vi "Append FFT block.vi"(8 "error in (no error)":errorcluster, 10 "new data":dbl[][](array[numeric]), 11 "ScopeBase in":refnum<class "ScopeBase.lvclass">) -> (0 "error out":errorcluster, 2 "FFT buffer":dbl[][](array[numeric]), 3 "ScopeBase out":refnum<class "ScopeBase.lvclass">)   [LabVIEW 2018, in "ScopeBase.lvclass"]
uses:
  ScopeBase.lvclass
  ScopeBase.lvclass/ScopeBase.ctl
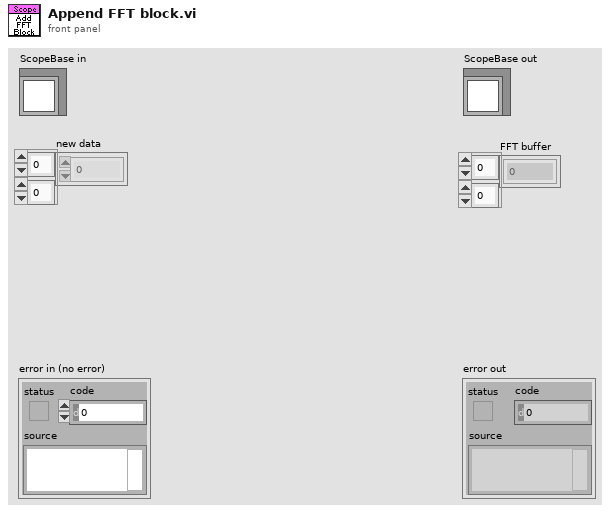
[diagram p1: front panel]
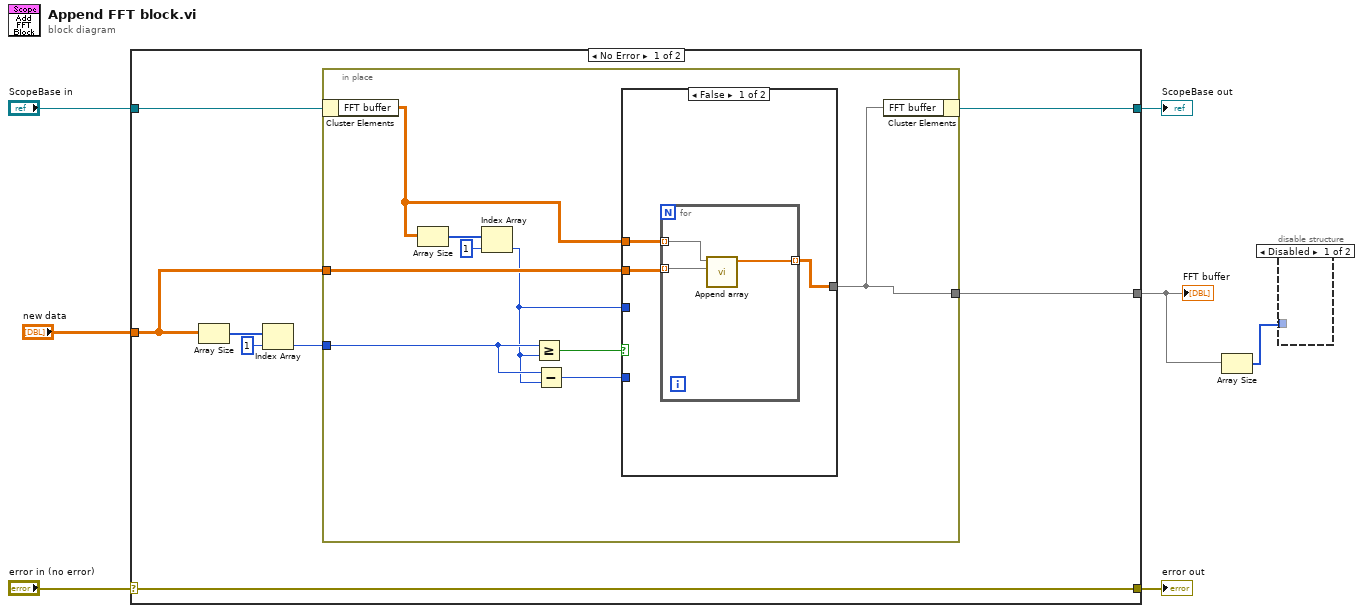
[diagram p0: block diagram]
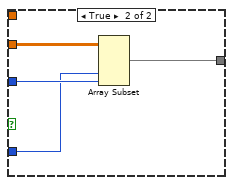
[diagram p3: hidden frame]
diagram:
  n1 = case shown="No Error" "error in (no error)" {
    selector: "error in (no error)" -> [w15 w36]
    tunnel: [w15 w36] -> w6
    tunnel: [w10 w35] -> w4
    tunnel: "ScopeBase in" -> [w13 w35]
    tunnel: "new data" -> [w9 _]
    tunnel: [w8 _] -> w2
    frame No Error {
      n2 = Array Size(array=w9) -> (size(s)=w14:i32[])
      n3 = Index Array(array=w14, index=1) -> (element=w11:i32)
      n4 = in-place {
        in-place-border: w11 -> [w20]
        in-place-border: w9 -> [w21]
        in-place-border: [w16] -> w8
        n5 = in-place-cluster #1(w13) -> ("FFT buffer"=w17:dbl[][])
        n6 = Array Size(array=w17) -> (size(s)=w24:i32[])
        n7 = Index Array(array=w24, index=1) -> (element=w19:i32)
        n8 = Greater Or Equal?(x=w20, y=w19) -> (x >= y?=w22:bool)
        n9 = Subtract(x=w20, y=w19) -> (x-y=w18:i32)
        n10 = case shown="False" w22 {
          tunnel: w21 -> [w27 w34]
          tunnel: w19 -> [_ w33]
          tunnel: w18 -> [_ w32]
          tunnel: [w25 w31] -> w16
          tunnel: w17 -> [w26 _]
          frame False {
            n11 = for {
              tunnel: w27 -> [w30] mode=indexing
              tunnel: w26 -> [w29] mode=indexing
              tunnel: [w28] -> w25 mode=indexing
              n12 = call "Append array.vi"("new section"=w30, "Array"=w29) -> ("Array 2"=w28:dbl[])  [unwired: 9 in]
            }
          }
          frame True {
            n13 = Array Subset(array=w34, index (col)=w32, length (col)=w33) -> (w31:dbl[][])  [unwired: 2 in]
          }
        }
        n14 = in-place-cluster #1("FFT buffer"=w16) -> (w10:refnum<class "ScopeBase.lvclass">)
      }
    }
    frame Error {
    }
  }
  "error out" <- w6
  "ScopeBase out" <- w4
  "FFT buffer" <- w2
  n15 = Array Size(array=w2) -> (size(s)=w1:i32[])
  n16 = disable-structure shown="Disabled" {
    disable-tunnel: w1 -> [_ _]
    frame Disabled {
    }
    frame Enabled {
    }
  }
